vi "Handle Notification.vi"(8 "error in (no error)":errorcluster, 9 "Payload":string, 10 "Notification Type":string, 11 "AI Assistant Template in":refnum<class "Configure Visa Device Channels.lvclass">) -> (0 "error out":errorcluster, 3 "AI Assistant Template out":refnum<class "Configure Visa Device Channels.lvclass">)   [LabVIEW 2026, in "Configure Visa Device Channels.lvlib" / "Configure Visa Device Channels.lvclass"]
uses:
  Configure Visa Device Channels.lvclass
  <vilib>/FlexLogger/SDK/PluginSDK.lvlibp/PEFClasses/SDK/Plugin/Plugin.lvclass
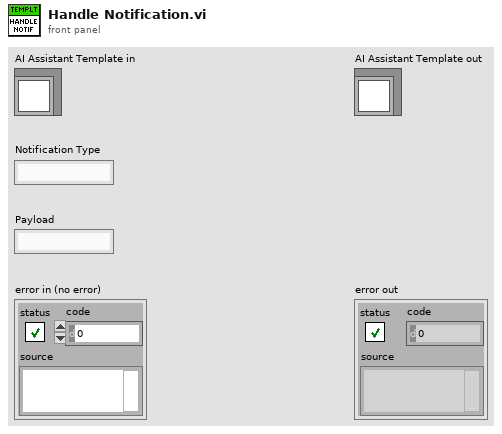
[diagram p1: front panel]
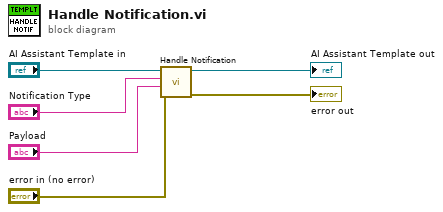
[diagram p0: block diagram]
diagram:
  n1 = call-parent "Handle Notification.vi"("error in (no error)"="error in (no error)", "Payload"="Payload", "Notification Type"="Notification Type", "Plugin in"="AI Assistant Template in") -> ("error out"=→"error out":errorcluster, "Plugin out"=→"AI Assistant Template out":refnum<class "Configure Visa Device Channels.lvclass">)  [unwired: 6 in]
